vi "Which_Trav_Setup.vi"(0 "Extra Command String":string, 1 "Input Position":sgl[](array[numeric])=[0.0, 0.0, 0.0] format="%.2f") -> (2 "Traverse Setups":string[](array[string]), 3 "XYZ Offset of 2nd Traverse":sgl[](array[numeric]), 4 "Traverse Positions":sgl[][](array[numeric]) format="%.2f")   [LabVIEW 2015]
uses:
  Globals/Extra_Commands_Global.vi
  Globals/Trav_pos_global.vi
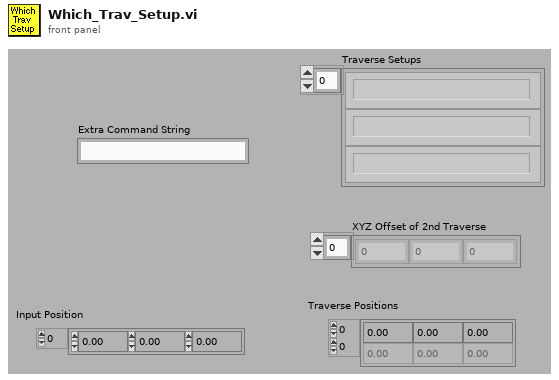
[diagram p1: front panel]
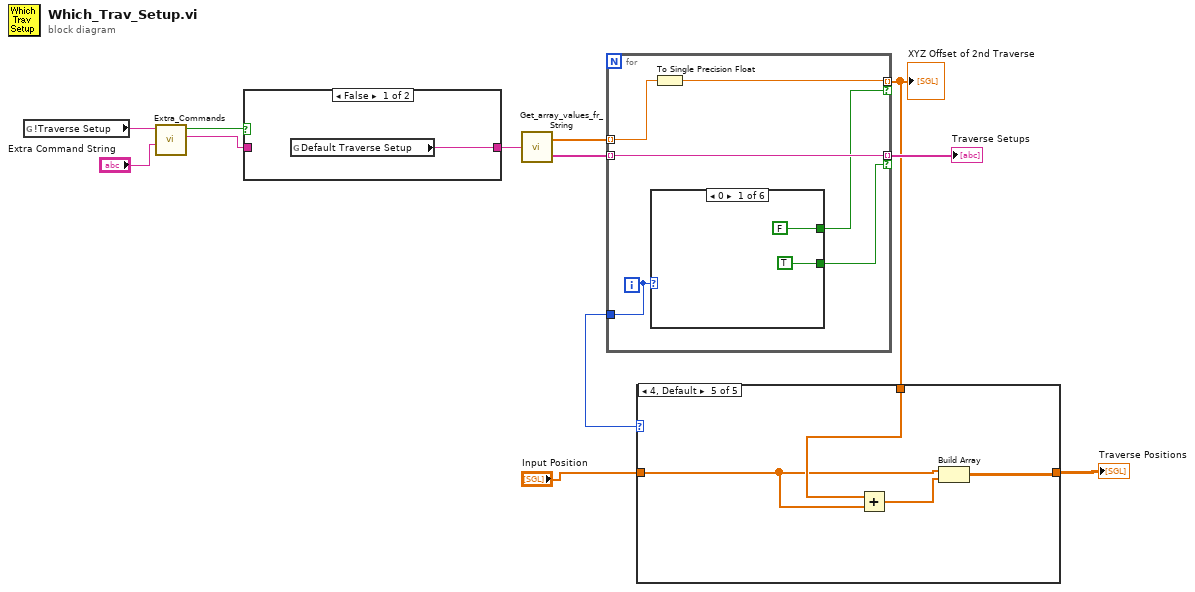
[diagram p0: block diagram]
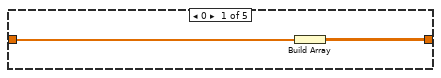
[diagram p2: hidden frame]
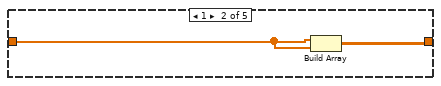
[diagram p3: hidden frame]
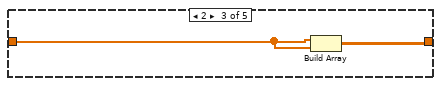
[diagram p4: hidden frame]
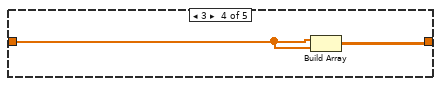
[diagram p5: hidden frame]
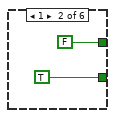
[diagram p6: hidden frame]
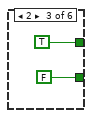
[diagram p7: hidden frame]
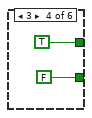
[diagram p8: hidden frame]
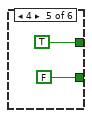
[diagram p9: hidden frame]
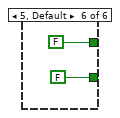
[diagram p10: hidden frame]
diagram:
  n1 = global read "Extra_Commands_Global.vi" "!Traverse Setup"() -> (w10:string)
  n2 = call "Extra_Commands.vi"("String to Search"="Extra Command String", "Command"=w10) -> ("String Value"=w12:string, "Command Found"=w11:bool)  [unwired: 1 in, 3 out]
  n3 = case shown="False" w11 {
    tunnel: [w13 w14] -> w8
    tunnel: w12 -> [_ w14]
    frame False {
      n4 = global read "Trav_pos_global.vi" "Default Traverse Setup"() -> (w13:string)
    }
    frame True {
    }
  }
  n5 = call "Get_array_values_fr_String.vi"("String Value"=w8) -> ("Numeric Array"=w5:dbl[], "String array"=w7:string[])
  n6 = for {
    tunnel: w7 -> [w20] mode=indexing
    tunnel: [w20] -> w6 mode=indexing if=w19
    tunnel: [w15] -> w1 mode=indexing if=w17
    tunnel: w5 -> [w18] mode=indexing
    tunnel: [w16] -> w4
    i -> [w16]
    n7 = case shown="0" w16 {
      tunnel: [TRUE TRUE FALSE FALSE FALSE FALSE] -> w19
      tunnel: [FALSE FALSE TRUE TRUE TRUE FALSE] -> w17
      frame 0 {
      }
      frame 1 {
      }
      frame 2 {
      }
      frame 3 {
      }
      frame 4 {
      }
      frame 5, Default {
      }
    }
    n8 = To Single Precision Float(number=w18) -> (single precision float=w15:sgl)
  }
  "Traverse Setups" <- w6
  "XYZ Offset of 2nd Traverse" <- w1
  n9 = case shown="4, Default" w4 {
    tunnel: "Input Position" -> [w34 w36 w38 w40 w42]
    tunnel: [w33 w35 w37 w39 w44] -> w2
    tunnel: w1 -> [_ _ _ _ w43]
    frame 0 {
      n10 = Build Array(w34) -> (w33:sgl[][])
    }
    frame 1 {
      n11 = Build Array(w36, w36) -> (w35:sgl[][])
    }
    frame 2 {
      n12 = Build Array(w38, w38) -> (w37:sgl[][])
    }
    frame 3 {
      n13 = Build Array(w40, w40) -> (w39:sgl[][])
    }
    frame 4, Default {
      n14 = Add(x=w43, y=w42) -> (x+y=w41:sgl[])
      n15 = Build Array(w42, w41) -> (w44:sgl[][])
    }
  }
  "Traverse Positions" <- w2
